vi "read big txt - rev1.vi"() -> (2 "selected path":path caption="선택된 경로", 3 "배열":string[](array[string]))   [LabVIEW 2015]
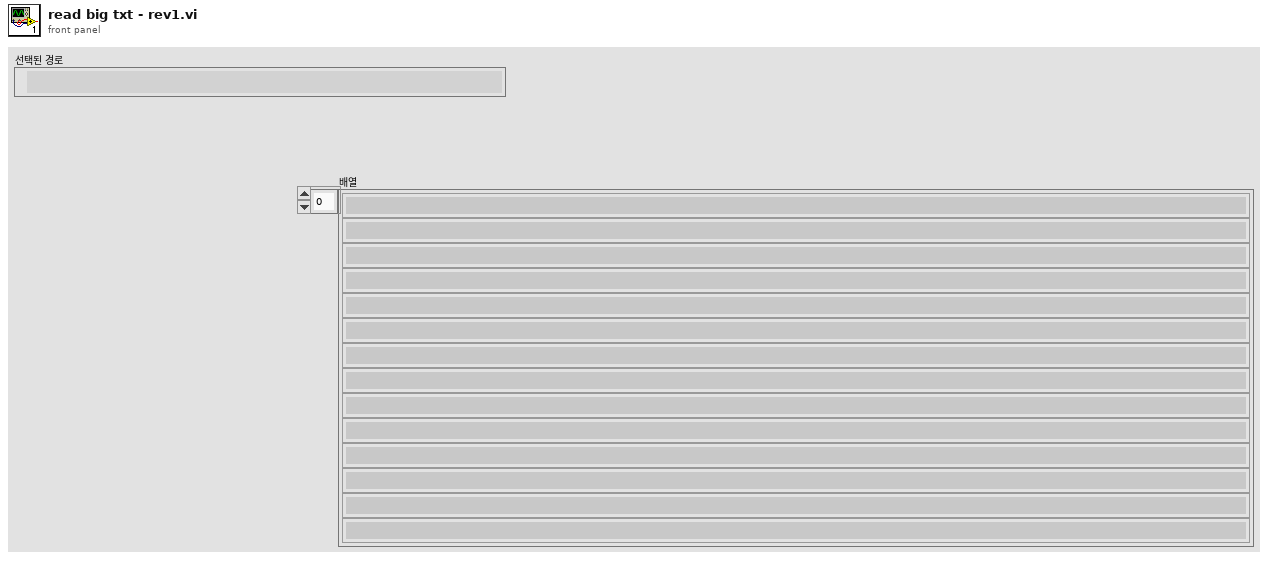
[diagram p1: front panel]
types:
  T1 = enum16{"open", "replace", "create", "open or create", "replace or create", "replace or create with confirmation"}
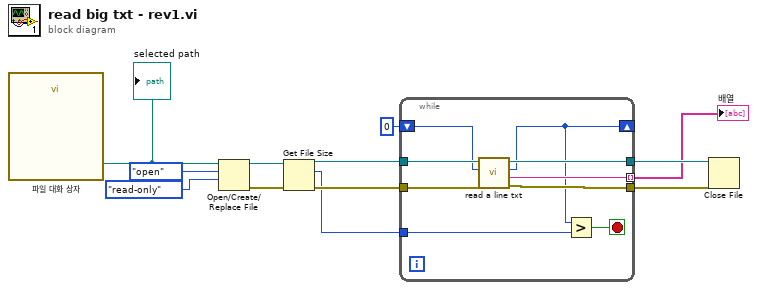
[diagram p0: block diagram]
diagram:
  n1 = call "파일 대화 상자"() -> ("selected path"=w12:path)  [unwired: 12 in, 3 out]
  "selected path" <- w12
  n2 = Open/Create/Replace File(file path (use dialog)=w12, operation (0:open)=T1."open" ("동작(0:open)"), access (0:read/write)=enum16{"read/write", "read-only", "write-only"}."read-only" ("접근(0:읽기/쓰기)")) -> (refnum out=w9:refnum<file>, error out=w8:errorcluster)  [unwired: 3 in, 1 out]
  n3 = Get File Size(file=w9, error in=w8) -> (refnum out=w7:refnum<file>, size (in bytes)=w1:i64, 0:w6:errorcluster)
  n4 = while {
    tunnel: [w21] -> w2 mode=indexing
    tunnel: w7 -> [w20]
    tunnel: w6 -> [w19]
    tunnel: [w18] -> w4
    tunnel: [w17] -> w3
    shift-right: [w15] -> _
    shift-left: i64 0 ("last offset+1") -> [w16]
    tunnel: w1 -> [w13]
    stop <- w14 stop-if-true
    n5 = call "read a line txt.vi"("에러 입력"=w19, "오프셋(바이트) (0)"=w16, "참조 번호"=w20) -> ("error out"=w17:errorcluster, "문자열"=w21:string, "last offset"=w15:i64, "refnum out"=w18:refnum<file>)  [unwired: 5 in]
    n6 = Greater?(x=w15, y=w13) -> (0:w14:bool)
  }
  "배열" <- w2
  n7 = Close File(refnum=w4, error in=w3) -> ()  [unwired: 2 out]
